vi "brc_daq_scan_modules.vi"() -> (14 "module_number":i32, 19 "error out":errorcluster)   [LabVIEW 2019, in "BRC-DAQ.lvlib"]
uses:
  BRC-DAQ.lvlib
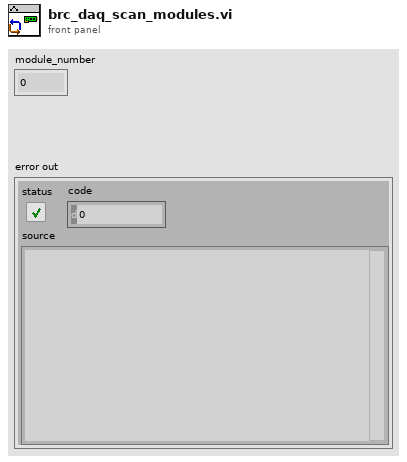
[diagram p1: front panel]
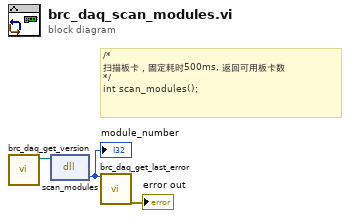
[diagram p0: block diagram]
diagram:
  # "/*\n扫描板卡，固定耗时500ms, 返回可用板卡数\n*/\nint scan_modules();"
  n1 = call "brc_daq_get_version.vi"() -> ("dll path"=w1:path)  [unwired: 11 in]
  n2 = dll-call lib="E:/01 BRC project/04BRC-daq/04 Drive/DAQ-x64/DLL/brc_daq_sdk.dll" fn="scan_modules"(path in=w1) -> ("return type"=w3:i32)  [unwired: 2 in, 2 out]
  "module_number" <- w3
  n3 = call "brc_daq_get_last_error.vi"("return_value"=w3) -> ("error out"=→"error out":errorcluster)  [unwired: 18 in]
